vi "KundtsTube2-week7J&J.vi"() -> ()   [LabVIEW 2015]
uses:
  <vilib>/Analysis/2dsp.llb/Real FFT.vi
  <vilib>/Analysis/NI_AALPro.lvlib
panel:
  out "?":cdb[](graph)
  out "FFT Graph":cdb[](graph)
  in  "stop":bool
  in  "Time (s)":dbl
  in  "Rate":dbl
  in  "Averages":dbl
  out "Results":T1
  out "Resonance Curve":cluster{"all rows":dbl[], "Array":dbl[]}[](graph)
  in  "Tab Control":enum32{"Simulation", "Experiment"}(tab)
  in  "Input Parameter":T2
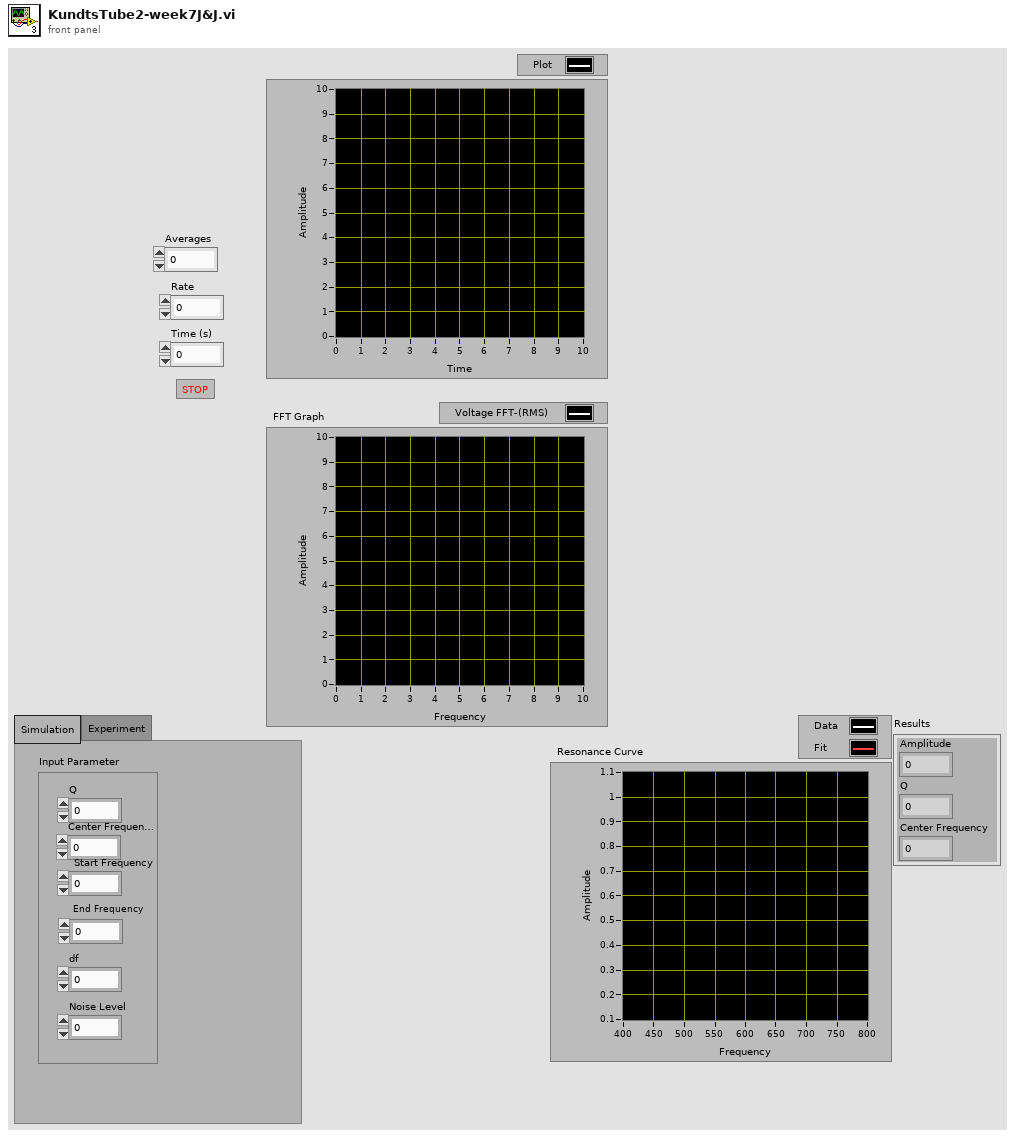
[diagram p1: front panel]
types:
  T1 = cluster{"Amplitude":dbl, "Q":dbl, "Center Frequency":dbl}
  T2 = cluster{"Q":dbl, "Center Frequency":dbl, "Start Frequency":dbl, " End Frequency":dbl, "df":dbl, "Noise Level":dbl}
  T3 = enum16{"open", "replace", "create", "open or create", "replace or create", "replace or create with confirmation"}
  T4 = cluster{"Resonance Curve[0]":cluster{"all rows":dbl[], "Array":dbl[]}, "Resonance Curve[1]":cluster{"all rows":dbl[], "Array":dbl[]}, "Resonance Curve[2]":cluster{"all rows":dbl[], "Array":dbl[]}, "Resonance Curve[3]":cluster{"all rows":dbl[], "Array":dbl[]}, "Resonance Curve[4]":cluster{"all rows":dbl[], "Array":dbl[]}, "Resonance Curve[5]":cluster{"all rows":dbl[], "Array":dbl[]}, "Resonance Curve[6]":cluster{"all rows":dbl[], "Array":dbl[]}, "Resonance Curve[7]":cluster{"all rows":dbl[], "Array":dbl[]}, "Resonance Curve[8]":cluster{"all rows":dbl[], "Array":dbl[]}}
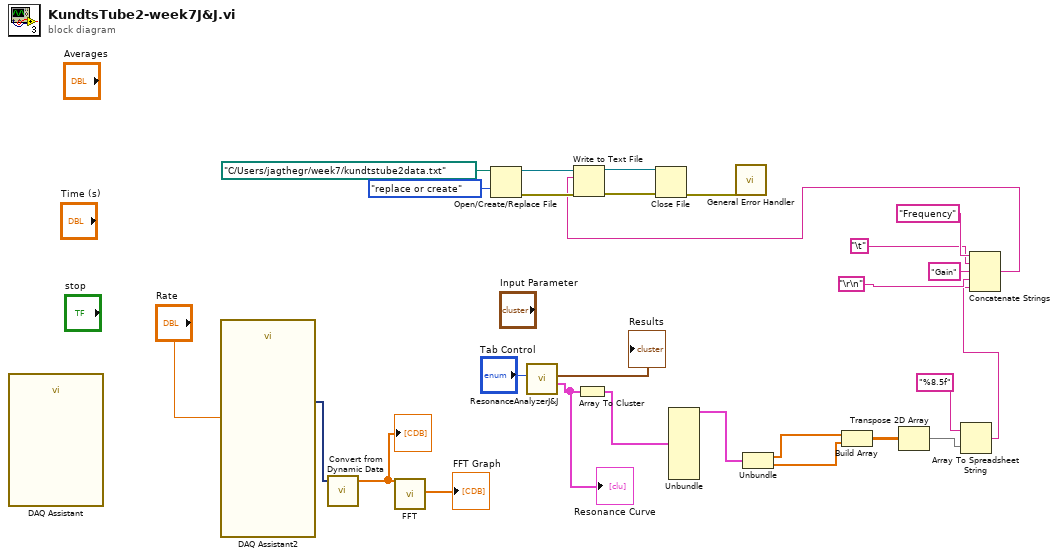
[diagram p0: block diagram]
diagram:
  n1 = call "DAQ Assistant"() -> ()  [unwired: 18 in, 2 out]
  n2 = call "DAQ Assistant2"("rate"="Rate") -> ("data"=w2:dynamicdata)  [unwired: 16 in, 2 out]
  n3 = call "Convert from Dynamic Data"("Dynamic Data Type"=w2) -> ("Array"=w1:dbl[])  [unwired: 3 in]
  "?" <- w1
  n4 = call-poly <vilib>:"FFT.vi"("X"=w1) -> ("FFT {X}"=→"FFT Graph":cdb[])  [unwired: 9 in, 1 out]
  n5 = Open/Create/Replace File(file path (use dialog)=path "C:/Users/jagthegr/week7/kundtstube2data.txt", operation (0:open)=T3."replace or create") -> (refnum out=w21:refnum<file>, error out=w22:errorcluster)  [unwired: 4 in, 1 out]
  n6 = call "ResonanceAnalyzerJ&J.vi"("Tab Control"="Tab Control") -> ("Resonance Curve"=w11:cluster{"all rows":dbl[], "Array":dbl[]}[], "Results"=→"Results":T1)  [unwired: 9 in]
  "Resonance Curve" <- w11
  n7 = Array To Cluster(array=w11) -> (cluster=w10:T4)
  n8 = Unbundle(w10) -> ("Resonance Curve[0]"=w9:cluster{"all rows":dbl[], "Array":dbl[]})  [unwired: 8 out]
  n9 = Unbundle(w9) -> ("all rows"=w8:dbl[], "Array"=w7:dbl[])
  n10 = Build Array(w8, w7) -> (w6:dbl[][])
  n11 = Transpose 2D Array(2D array=w6) -> (transposed array=w5:dbl[][])
  n12 = Array To Spreadsheet String(array=w5, 3:"%8.5f" ("format string")) -> (spreadsheet string=w13:string)  [unwired: 1 in]
  n13 = Concatenate Strings("Frequency" ("string"), "\t", "Gain" ("string"), "\r\n", w13) -> (w12:string)
  n14 = Write to Text File(file (use dialog)=w21, text=w12, error in=w22) -> (refnum out=w20:refnum<file>, error out=w23:errorcluster)  [unwired: 1 in, 1 out]
  n15 = Close File(refnum=w20, error in=w23) -> (error out=w24:errorcluster)  [unwired: 1 out]
  n16 = call <vilib>:"General Error Handler.vi"("error in (no error)"=w24) -> ()  [unwired: 10 in, 5 out]
